vi "Read iRFRaw.vi"(8 "error in (no error)":errorcluster, 11 "APDClass in":refnum<class "APDClass.lvclass">) -> (0 "error out":errorcluster, 2 "iRFRaw":cluster{"CtrlV":dbl, "WFs":dbl[][]}[](array[cluster]), 3 "APDClass out":refnum<class "APDClass.lvclass">)   [LabVIEW 2020, in "APDClass.lvclass"]
uses:
  APDClass.lvclass
  APDClass.lvclass/APDClass.ctl
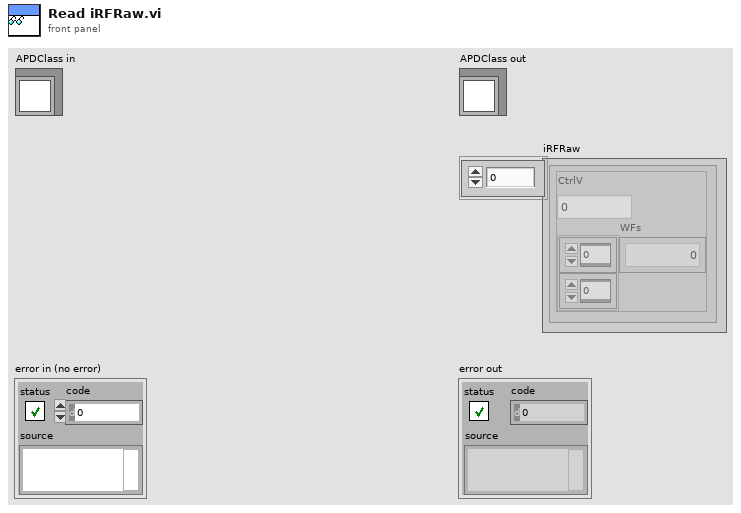
[diagram p1: front panel]
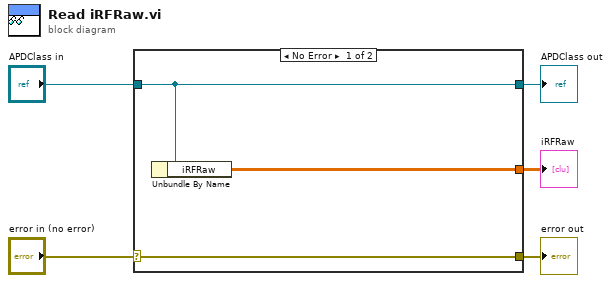
[diagram p0: block diagram]
diagram:
  n1 = case shown="No Error" "error in (no error)" {
    selector: "error in (no error)" -> [w8 w9]
    tunnel: [w8 w9] -> w4
    tunnel: [w7 w10] -> w2
    tunnel: "APDClass in" -> [w7 w10]
    tunnel: [w6 _] -> w1
    frame No Error {
      n2 = Unbundle By Name(w7) -> ("iRFRaw"=w6:dbl[][])
    }
    frame Error {
    }
  }
  "error out" <- w4
  "APDClass out" <- w2
  "iRFRaw" <- w1
